vi "SET_COMPENSATION_n.vi"(2 "execute":bool, 5 "measure COMP value":bool, 9 "COMPENSATION":bool, 11 "error in (no error)":errorcluster) -> (4 "function return":string, 15 "error out":errorcluster)   [LabVIEW 2017, in "ZBOX_IS.lvlib"]
uses:
  ZBOX_IS.lvlib
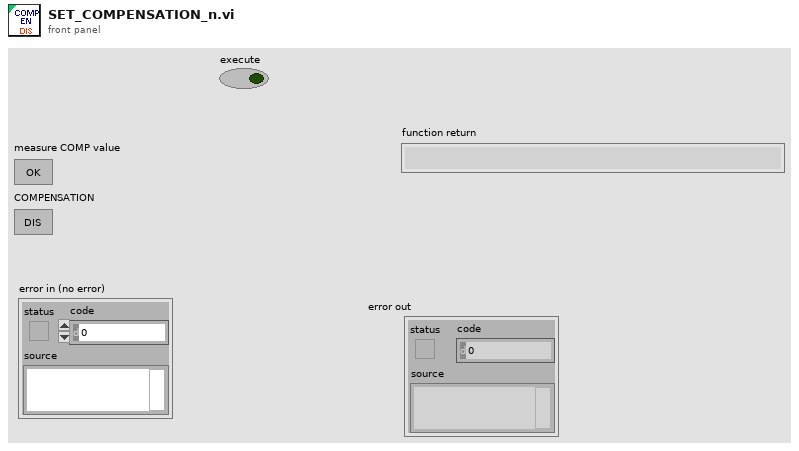
[diagram p1: front panel]
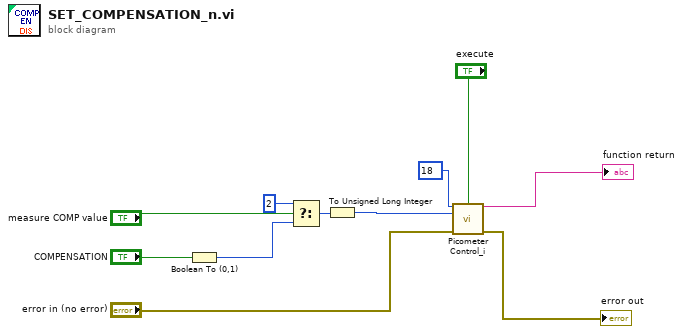
[diagram p0: block diagram]
diagram:
  n1 = Boolean To (0,1)(Boolean="COMPENSATION") -> (0, 1=w3:i16)
  n2 = Select(t=u32 2, s="measure COMP value", f=w3) -> (s? t:f=w5:u32)
  n3 = To Unsigned Long Integer(number=w5) -> (unsigned 32bit integer=w2:u32)
  n4 = call "Picometer Control_i.vi"("Cmd"=u8 18, "execute"="execute", "ulValue"=w2, "error in (no error)"="error in (no error)") -> ("function return"=→"function return":string, "error out"=→"error out":errorcluster)  [unwired: 7 in, 3 out]
